vi "documentFactory (by Type).vi"(8 "error in (no error)":errorcluster, 11 "Document Type":T1) -> (0 "error out":errorcluster, 3 "npoiDocument out":refnum<class "npoiDocument.lvclass">)   [LabVIEW 2017, in "Document API.lvlib" / "Document API.lvclass"]
uses:
  Document API.lvclass
  NPOI_Document/npoiDocument/npoiDocument.lvclass
  Document Type.ctl
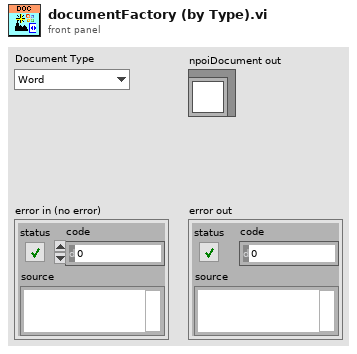
[diagram p1: front panel]
types:
  T1 = typedef "Document API.lvlib/Document API.lvclass/Document Type.ctl" = enum16{"Word", "Excel"}
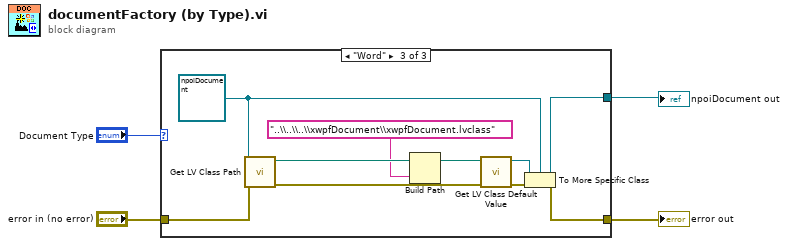
[diagram p0: block diagram]
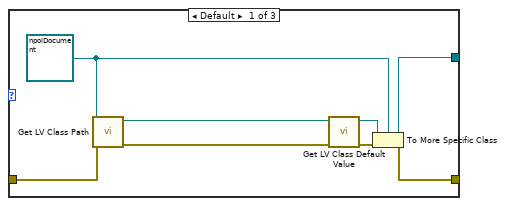
[diagram p2: hidden frame]
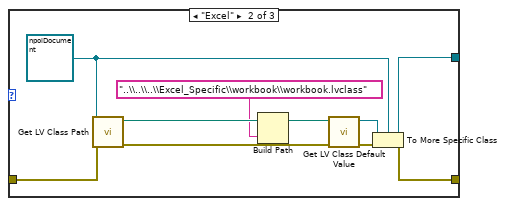
[diagram p3: hidden frame]
diagram:
  n1 = case shown="\"Word\"" "Document Type" {
    tunnel: [w12 w22 w32] -> w3
    tunnel: "error in (no error)" -> [w11 w21 w31]
    tunnel: [w10 w20 w30] -> w4
    frame Default {
      w9 = refnum<class "npoiDocument.lvclass"> refnum ("NPOI_Document.lvlib:npoiDocument.lvclass")
      n2 = call <vilib>:"Get LV Class Path.vi"("error in (no error)"=w11, "object"=w9) -> ("error out"=w8:errorcluster, "class path"=w7:path)  [unwired: 8 in]
      n3 = call <vilib>:"Get LV Class Default Value.vi"("error in (no error)"=w8, "class path"=w7) -> ("error out"=w6:errorcluster, "object"=w5:refnum<class>)  [unwired: 8 in]
      n4 = To More Specific Class(target class=w9, reference=w5, error in=w6) -> (specific class reference=w12:refnum<class "npoiDocument.lvclass">, error out=w10:errorcluster)
    }
    frame "Excel" {
      w19 = refnum<class "npoiDocument.lvclass"> refnum ("NPOI_Document.lvlib:npoiDocument.lvclass")
      n5 = call <vilib>:"Get LV Class Path.vi"("error in (no error)"=w21, "object"=w19) -> ("error out"=w18:errorcluster, "class path"=w17:path)  [unwired: 8 in]
      n6 = Build Path(base path=w17, name or relative path="..\\..\\..\\Excel_Specific\\workbook\\workbook.lvclass") -> (appended path=w14:path)
      n7 = call <vilib>:"Get LV Class Default Value.vi"("error in (no error)"=w18, "class path"=w14) -> ("error out"=w16:errorcluster, "object"=w15:refnum<class>)  [unwired: 8 in]
      n8 = To More Specific Class(target class=w19, reference=w15, error in=w16) -> (specific class reference=w22:refnum<class "npoiDocument.lvclass">, error out=w20:errorcluster)
    }
    frame "Word" {
      w29 = refnum<class "npoiDocument.lvclass"> refnum ("NPOI_Document.lvlib:npoiDocument.lvclass")
      n9 = call <vilib>:"Get LV Class Path.vi"("error in (no error)"=w31, "object"=w29) -> ("error out"=w28:errorcluster, "class path"=w27:path)  [unwired: 8 in]
      n10 = Build Path(base path=w27, name or relative path="..\\..\\..\\xwpfDocument\\xwpfDocument.lvclass") -> (appended path=w24:path)
      n11 = call <vilib>:"Get LV Class Default Value.vi"("error in (no error)"=w28, "class path"=w24) -> ("error out"=w26:errorcluster, "object"=w25:refnum<class>)  [unwired: 8 in]
      n12 = To More Specific Class(target class=w29, reference=w25, error in=w26) -> (specific class reference=w32:refnum<class "npoiDocument.lvclass">, error out=w30:errorcluster)
    }
  }
  "error out" <- w4
  "npoiDocument out" <- w3
